vi "Timing Statistics.vi"(11 "Execution Speeds":dbl[](array[numeric])) -> (3 "Timing Statistics":T1)   [LabVIEW 2020, in "slsc-switch-benchmarks.lvlib"]
uses:
  slsc-switch-benchmarks.lvlib
  Timing Statistics.ctl
  <vilib>/Analysis/NI_AALBase.lvlib
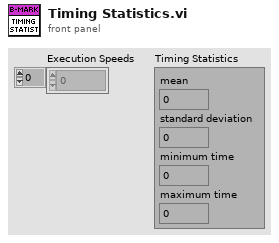
[diagram p1: front panel]
types:
  T1 = typedef "slsc-switch-benchmarks.lvlib/Timing Statistics.ctl" = cluster{"mean":dbl, "standard deviation":dbl, "minimum time":dbl, "maximum time":dbl}
  T2 = cluster{"mean":dbl, "standard deviation":dbl, dbl, dbl}
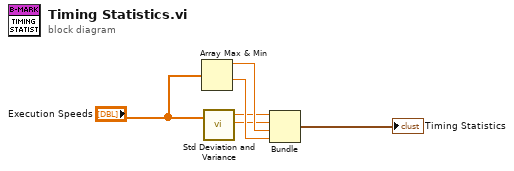
[diagram p0: block diagram]
diagram:
  n1 = Array Max & Min(array="Execution Speeds") -> (max value=w4:dbl, min value=w5:dbl)  [unwired: 2 out]
  n2 = call <vilib>:"Std Deviation and Variance.vi"("X"="Execution Speeds") -> ("mean"=w2:dbl, "standard deviation"=w3:dbl)  [unwired: 1 in, 1 out]
  n3 = Bundle("mean"=w2, "standard deviation"=w3, w4, w5) -> (→"Timing Statistics":T2)  [unwired: 1 in]
